vi "Drive Drive.vi"(1 "Drive Info In":T1) -> (0 "Drive Info Out":T1)   [LabVIEW 2013]
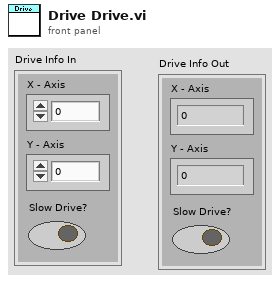
[diagram p1: front panel]
types:
  T1 = cluster{"X - Axis":dbl, "Y - Axis":dbl, "Slow Drive?":bool}
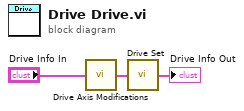
[diagram p0: block diagram]
diagram:
  n1 = call "Drive Axis Modifications.vi"("Drive Info In"="Drive Info In") -> ("Drive Info Out"=w2:T1)
  n2 = call "Drive Set.vi"("Drive Info In"=w2) -> ("Drive Info Out"=→"Drive Info Out":T1)
